vi "DevScripts_CreateWindowPropertyNamesComboBox.vi"() -> ()   [LabVIEW 2024]
uses:
  <vilib>/Utility/error.llb/Trim Whitespace One-Sided.vi
  SDL3/Video/WindowPropertyName--combobox.ctl
  SDL3/Video/Video.lvlib
panel:
  out "Array 2":string[](array[string])
  out "Array":string[](array[string])
  in  "#Define list":string="#define SDL_PROP_WINDOW_CREATE_ALWAYS_ON_TOP_BOOLEAN               \"SDL.window.create.always_on_top\"\n#define SDL_PROP_WINDOW_CREATE_BORDERLESS_BOOLEAN                  \"SDL.window.create.borderless\"\n#define SDL_PROP_WINDOW_CREATE_FOCUSABLE_BOOLEAN                   \"SDL.window.create.focusable\"\n#define SDL_PROP_WINDOW_CREATE_EXTERNAL_GRAPHICS_CONTEXT_BOOLEAN   \"SDL.window.create.external_graphics_context\"\n#define SDL_PROP_WINDOW_CREATE_FLAGS_NUMBER                        \"SDL.window.create.flags\"\n#define SDL_PROP_WINDOW_CREATE_FULLSCREEN_BOOLEAN                  \"SDL.window.create.fullscreen\"\n#define SDL_PROP_WINDOW_CREATE_HEIGHT_NUMBER                       \"SDL.window.create.height\"\n#define SDL_PROP_WINDOW_CREATE_HIDDEN_BOOLEAN                      \"SDL.window.create.hidden\"\n#define SDL_PROP_WINDOW_CREATE_HIGH_PIXEL_DENSITY_BOOLEAN          \"SDL.window.create.high_pixel_density\"\n#define SDL_PROP_WINDOW_CREATE_MAXIMIZED_BOOLEAN                   \"SDL.window.create.maximized\"\n#define SDL_PROP_WINDOW_CREATE_MENU_BOOLEAN                        \"SDL.window.create.menu\"\n#define SDL_PROP_WINDOW_CREATE_METAL_BOOLEAN                       \"SDL.window.create.metal\"\n#define SDL_PROP_WINDOW_CREATE_MINIMIZED_BOOLEAN                   \"SDL.window.create.minimized\"\n#define SDL_PROP_WINDOW_CREATE_MODAL_BOOLEAN                       \"SDL.window.create.modal\"\n#define SDL_PROP_WINDOW_CREATE_MOUSE_GRABBED_BOOLEAN               \"SDL.window.create.mouse_grabbed\"\n#define SDL_PROP_WINDOW_CREATE_OPENGL_BOOLEAN                      \"SDL.window.create.opengl\"\n#define SDL_PROP_WINDOW_CREATE_PARENT_POINTER                      \"SDL.window.create.parent\"\n#define SDL_PROP_WINDOW_CREATE_RESIZABLE_BOOLEAN                   \"SDL.window.create.resizable\"\n#define SDL_PROP_WINDOW_CREATE_TITLE_STRING                        \"SDL.window.create.title\"\n#define SDL_PROP_WINDOW_CREATE_TRANSPARENT_BOOLEAN                 \"SDL.window.create.transparent\"\n#define SDL_PROP_WINDOW_CREATE_TOOLTIP_BOOLEAN                     \"SDL.window.create.tooltip\"\n#define SDL_PROP_WINDOW_CREATE_UTILITY_BOOLEAN                     \"SDL.window.create.utility\"\n#define SDL_PROP_WINDOW_CREATE_VULKAN_BOOLEAN                      \"SDL.window.create.vulkan\"\n#define SDL_PROP_WINDOW_CREATE_WIDTH_NUMBER                        \"SDL.window.create.width\"\n#define SDL_PROP_WINDOW_CREATE_X_NUMBER                            \"SDL.window.create.x\"\n#define SDL_PROP_WINDOW_CREATE_Y_NUMBER                            \"SDL.window.create.y\"\n#define SDL_PROP_WINDOW_CREATE_COCOA_WINDOW_POINTER                \"SDL.window.create.cocoa.window\"\n#define SDL_PROP_WINDOW_CREATE_COCOA_VIEW_POINTER                  \"SDL.window.create.cocoa.view\"\n#define SDL_PROP_WINDOW_CREATE_WAYLAND_SURFACE_ROLE_CUSTOM_BOOLEAN \"SDL.window.create.wayland.surface_role_custom\"\n#define SDL_PROP_WINDOW_CREATE_WAYLAND_CREATE_EGL_WINDOW_BOOLEAN   \"SDL.window.create.wayland.create_egl_window\"\n#define SDL_PROP_WINDOW_CREATE_WAYLAND_WL_SURFACE_POINTER          \"SDL.window.create.wayland.wl_surface\"\n#define SDL_PROP_WINDOW_CREATE_WIN32_HWND_POINTER                  \"SDL.window.create.win32.hwnd\"\n#define SDL_PROP_WINDOW_CREATE_WIN32_PIXEL_FORMAT_HWND_POINTER     \"SDL.window.create.win32.pixel_format_hwnd\"\n#define SDL_PROP_WINDOW_CREATE_X11_WINDOW_NUMBER                   \"SDL.window.create.x11.window\""
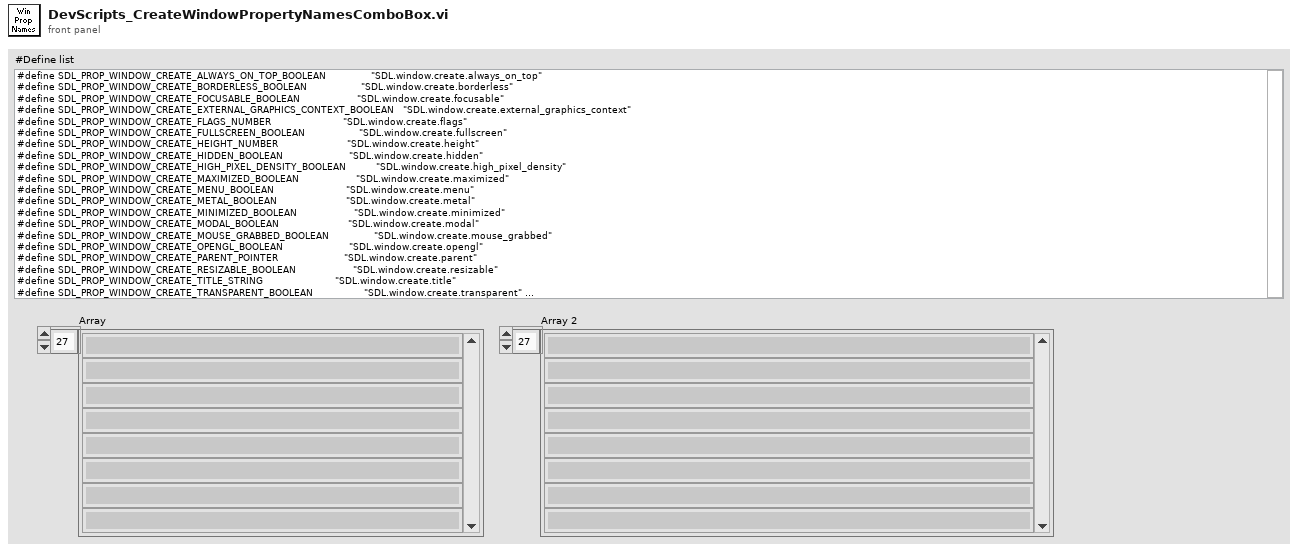
[diagram p1: front panel]
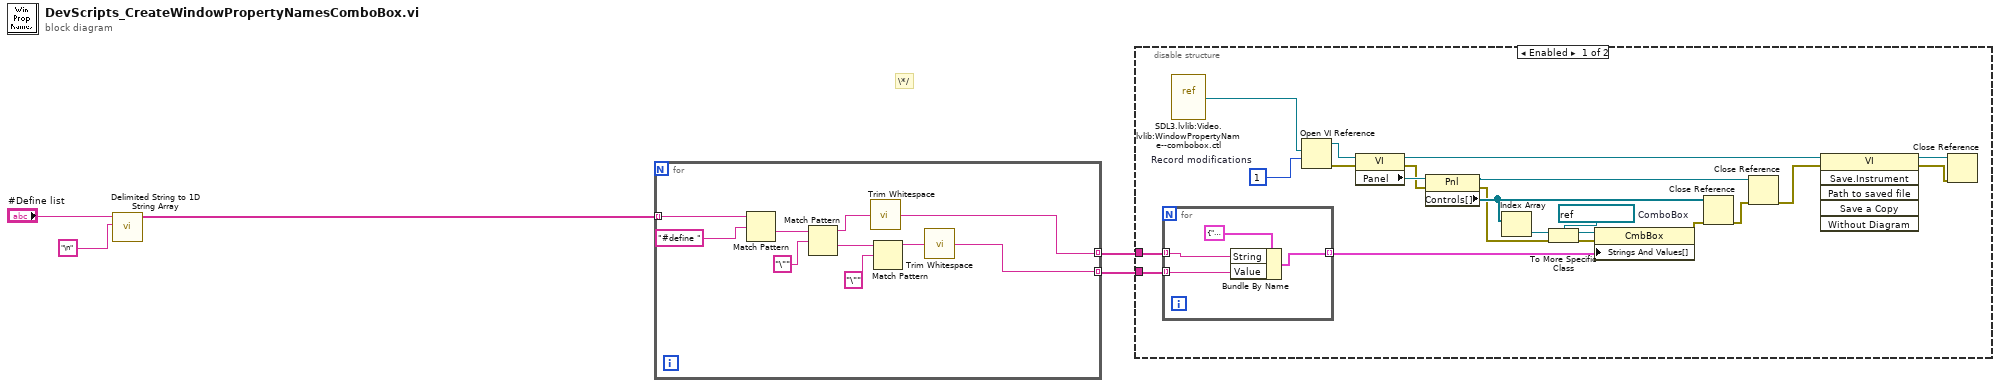
[diagram p0: block diagram]
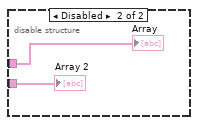
[diagram p2: hidden frame]
diagram:
  # "\\*/"
  n1 = call <vilib>:"Delimited String to 1D String Array.vi"("delimiter"="\n", "delimited string"="#Define list") -> ("string array"=w2:string[])  [unwired: 9 in]
  n2 = for {
    tunnel: w2 -> [w15] mode=indexing
    tunnel: [w8] -> w3 mode=indexing
    tunnel: [w6] -> w1 mode=indexing
    n3 = Match Pattern(string=w15, regular expression="#define ") -> (after substring=w13:string)  [unwired: 1 in, 3 out]
    n4 = Match Pattern(string=w13, regular expression="\"") -> (before substring=w7:string, after substring=w11:string)  [unwired: 1 in, 2 out]
    n5 = call <vilib>:"Trim Whitespace.vi"("string"=w7) -> ("trimmed string"=w8:string)  [unwired: 1 in]
    n6 = Match Pattern(string=w11, regular expression="\"") -> (before substring=w9:string)  [unwired: 1 in, 3 out]
    n7 = call <vilib>:"Trim Whitespace.vi"("string"=w9) -> ("trimmed string"=w6:string)  [unwired: 1 in]
  }
  n8 = disable-structure shown="Enabled" {
    disable-tunnel: w3 -> [w18 w43]
    disable-tunnel: w1 -> [w17 w42]
    frame Enabled {
      w29 = refnum<vi> refnum  # ComboBox
      w35 = 1  # Record modifications
      n9 = for {
        tunnel: w18 -> [w40] mode=indexing
        tunnel: w17 -> [w39] mode=indexing
        tunnel: [w38] -> w16 mode=indexing
        n10 = Bundle By Name(cluster=cluster{"String":string, "Value":string} {"String"="", "Value"=""}, "String"=w40, "Value"=w39) -> (w38:cluster{"String":string, "Value":string})
      }
      n11 = vi-ref "SDL3.lvlib:Video.lvlib:WindowPropertyName--combobox.ctl"() -> (w36:refnum<vi>)
      n12 = Open VI Reference(vi path=w36, options=w35) -> (vi reference=w34:refnum<vi>, error out=w37:errorcluster)  [unwired: 4 in]
      n13 = property class="VI"(reference=w34, error in=w37) -> (reference out=w24:refnum<vi>, error out=w32:errorcluster, "Panel"=w33:refnum<vi>)
      n14 = property class="Pnl"(reference=w33, error in=w32) -> (reference out=w31:refnum<vi>, error out=w22:errorcluster, "Controls[]"=w27:refnum<vi>[])
      n15 = Index Array(array=w27) -> (element=w28:refnum<vi>)  [unwired: 1 in]
      n16 = To More Specific Class(target class=w29, reference=w28, error in=w22) -> (specific class reference=w21:refnum<vi>, error out=w20:errorcluster)
      n17 = property class="CmbBox"(reference=w21, error in=w20, "Strings And Values[]"=w16) -> (error out=w19:errorcluster)  [unwired: 1 out]
      n18 = Close Reference(reference=w27, error in (no error)=w19) -> (error out=w26:errorcluster)
      n19 = Close Reference(reference=w31, error in (no error)=w26) -> (error out=w30:errorcluster)
      n20 = invoke class="VI" method="Save.Instrument"(reference=w24, error in=w30) -> (reference out=w23:refnum<vi>, error out=w25:errorcluster)  [unwired: 4 in, 4 out]
      n21 = Close Reference(reference=w23, error in (no error)=w25) -> ()  [unwired: 1 out]
    }
    frame Disabled {
      "Array" <- w43
      "Array 2" <- w42
    }
  }
